vi "Resistivity_engine.vi"(6 "I (A)":dbl=0.001, 7 "M":i32=1, 8 "error in":errorcluster, 9 "GPC (A/cycle)":dbl, 10 "N (cycle)":dbl, 11 "Keithley 4200 VISA":refnum<visa-resource-name>="TCPIP0::192.168.0.4::1225::SOCKET") -> (0 "error out":errorcluster, 2 "rho (uOhm*cm)":dbl, 3 "Rs out":string, 4 "valid?":bool, 5 "Rs (Ohm/sq)":dbl)   [LabVIEW 2026]
panel:
  out "thickness (nm)":dbl
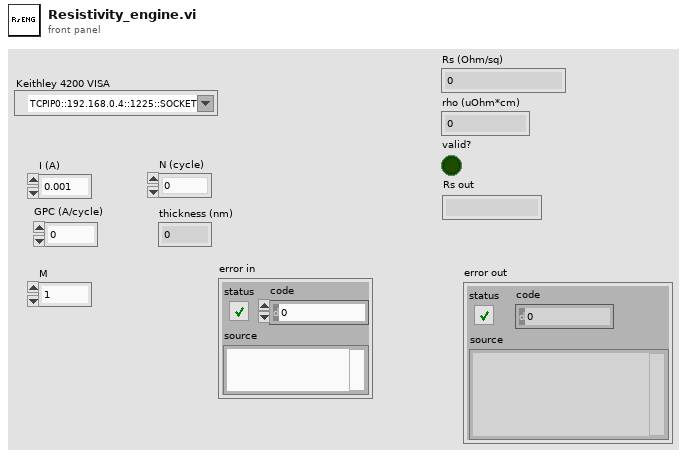
[diagram p1: front panel]
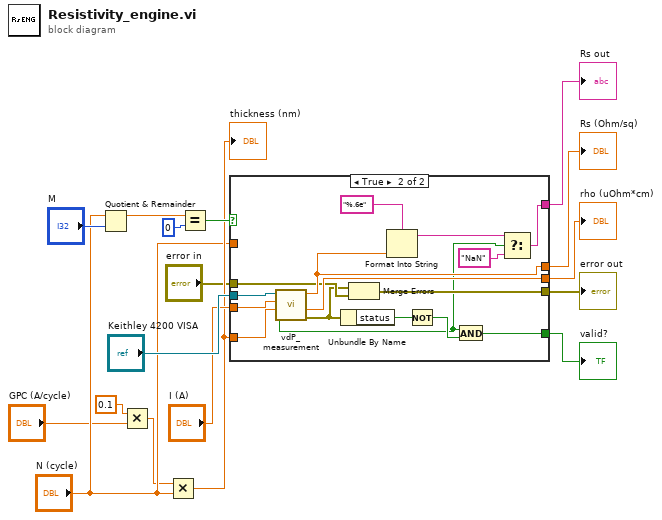
[diagram p0: block diagram]
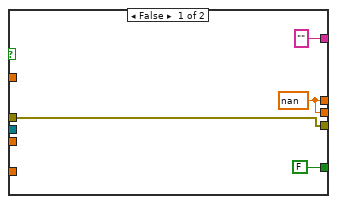
[diagram p2: hidden frame]
diagram:
  n1 = Quotient & Remainder(x="N (cycle)", y="M") -> (x-y*floor(x/y)=w14:dbl)  [unwired: 1 out]
  n2 = Multiply(x=0.1, y="GPC (A/cycle)") -> (x*y=w1:dbl)
  n3 = Multiply(x=w1, y="N (cycle)") -> (x*y=w11:dbl)
  "thickness (nm)" <- w11
  n4 = Equal?(x=w14, y=0) -> (x = y?=w12:bool)
  n5 = case shown="True" w12 {
    tunnel: w11 -> [_ w35]
    tunnel: "Keithley 4200 VISA" -> [_ w37]
    tunnel: "I (A)" -> [_ w36]
    tunnel: "N (cycle)" -> [_ _]
    tunnel: ["" w31] -> w7
    tunnel: [w20 w30] -> w9
    tunnel: [FALSE w22] -> w8
    tunnel: [w20 w29] -> w4
    tunnel: "error in" -> [w18 w28]
    tunnel: [w18 w27] -> w5
    frame False {
      w20 = nan
    }
    frame True {
      n6 = call "vdP_measurement.vi"("Thickness (nm)"=w35, "Source Current (A)"=w36, "VISA resource name"=w37) -> ("error out"=w26:errorcluster, "rho (uOhm * cm)"=w29:dbl, "Rs (Ohm/sq)"=w30:dbl, "Valid?"=w23:bool)  [unwired: 2 in]
      n7 = Unbundle By Name(w26) -> ("status"=w25:bool)
      n8 = Merge Errors(w26, w28) -> (w27:errorcluster)
      n9 = Format Into String(format string="%.6e", w30) -> (resulting string=w33:string)  [unwired: 2 in, 1 out]
      n10 = Not(x=w25) -> (.not. x?=w24:bool)
      n11 = And(x=w23, y=w24) -> (x .and. y?=w22:bool)
      n12 = Select(t=w33, s=w23, f="NaN") -> (s? t:f=w31:string)
    }
  }
  "Rs (Ohm/sq)" <- w9
  "rho (uOhm*cm)" <- w4
  "valid?" <- w8
  "Rs out" <- w7
  "error out" <- w5
